vi "SW_Get_passw_hash.vi"(2 "Password":string, 3 "Username":string) -> (0 "Password hash":string, 1 "Username":string)   [LabVIEW 2016]
uses:
  <userlib>/_OpenG.lib/md5/md5.llb/MD5 Message Digest (Hexadecimal String)__ogtk.vi
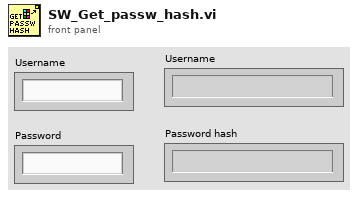
[diagram p1: front panel]
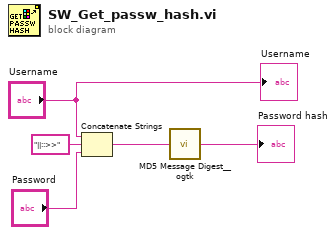
[diagram p0: block diagram]
diagram:
  n1 = Concatenate Strings("Username", "||::>>" ("string"), "Password") -> (w3:string)
  n2 = call-poly <userlib>:"MD5 Message Digest__ogtk.vi"("Message"=w3) -> ("MD5 Message Digest"=→"Password hash":string)
  "Username" <- "Username"
